vi "Tolerance to color convert.vi"() -> ()   [LabVIEW 2018]
uses:
  Tolerance.ctl
  Resistor Band Colors.lvlib
panel:
  in  "Tolerance":T1
  out "Color":u32
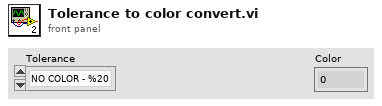
[diagram p1: front panel]
types:
  T1 = typedef "Tolerance.ctl" = enum16{"NO COLOR - %20", "Brown - %1", "Red - %2", "Orange - %3", "Yellow - %4", "Green - %0,5", "Blue - %0,25", "Violet - %0,10", "Grey - %0,05", "Silver x - %10", "Gold x - %5"}
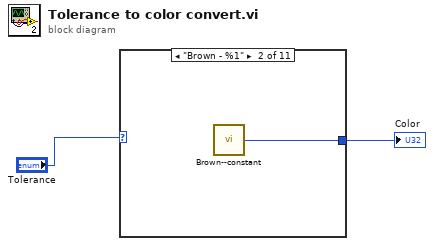
[diagram p0: block diagram]
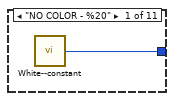
[diagram p2: hidden frame]
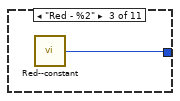
[diagram p3: hidden frame]
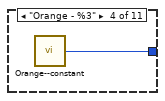
[diagram p4: hidden frame]
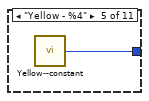
[diagram p5: hidden frame]
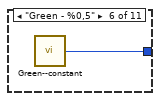
[diagram p6: hidden frame]
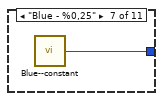
[diagram p7: hidden frame]
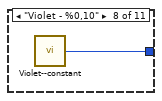
[diagram p8: hidden frame]
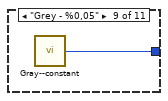
[diagram p9: hidden frame]
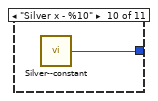
[diagram p10: hidden frame]
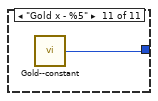
[diagram p11: hidden frame]
diagram:
  n1 = case shown="\"Brown - %1\"" "Tolerance" {
    tunnel: [w3 w4 w5 w6 w7 w8 w9 w10 w11 w12 w13] -> w2
    frame "NO COLOR - %20" {
      n2 = call "White--constant.vi"() -> ("Color"=w3:u32)  [unwired: 5 in]
    }
    frame "Brown - %1" {
      n3 = call "Brown--constant.vi"() -> ("Color"=w4:u32)  [unwired: 5 in]
    }
    frame "Red - %2" {
      n4 = call "Red--constant.vi"() -> ("Color"=w5:u32)  [unwired: 5 in]
    }
    frame "Orange - %3" {
      n5 = call "Orange--constant.vi"() -> ("Color"=w6:u32)  [unwired: 5 in]
    }
    frame "Yellow - %4" {
      n6 = call "Yellow--constant.vi"() -> ("Color"=w7:u32)  [unwired: 5 in]
    }
    frame "Green - %0,5" {
      n7 = call "Green--constant.vi"() -> ("Color"=w8:u32)  [unwired: 5 in]
    }
    frame "Blue - %0,25" {
      n8 = call "Blue--constant.vi"() -> ("Color"=w9:u32)  [unwired: 5 in]
    }
    frame "Violet - %0,10" {
      n9 = call "Violet--constant.vi"() -> ("Color"=w10:u32)  [unwired: 5 in]
    }
    frame "Grey - %0,05" {
      n10 = call "Gray--constant.vi"() -> ("Color"=w11:u32)  [unwired: 5 in]
    }
    frame "Silver x - %10" {
      n11 = call "Silver--constant.vi"() -> ("Color"=w12:u32)  [unwired: 5 in]
    }
    frame "Gold x - %5" {
      n12 = call "Gold--constant.vi"() -> ("Color"=w13:u32)  [unwired: 5 in]
    }
  }
  "Color" <- w2
